vi "Sequence Create PDA Column.vi"(8 "error in (no error)":errorcluster, 11 "Connection Refnum":T1) -> (0 "error out":errorcluster, 3 "Connection Refnum":T1)   [LabVIEW 2011]
uses:
  SI.LIB/ODBC/SQL Controls/Connection Refnum.ctl
panel:
  out "Possible error out":errorcluster
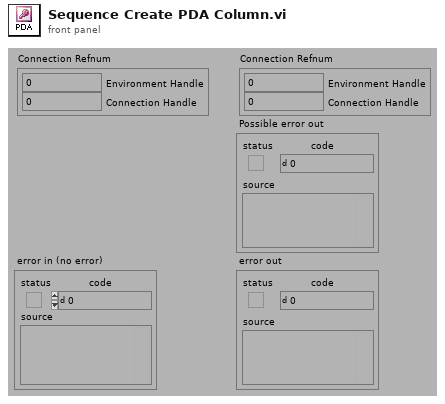
[diagram p1: front panel]
types:
  T1 = typedef "Connection Refnum.ctl" = cluster{"Environment Handle":i32, "Connection Handle":i32}
  T2 = typedef "Statement Refnum.ctl" = cluster{"Statement Handle":i32, "Parameter Number":u16}
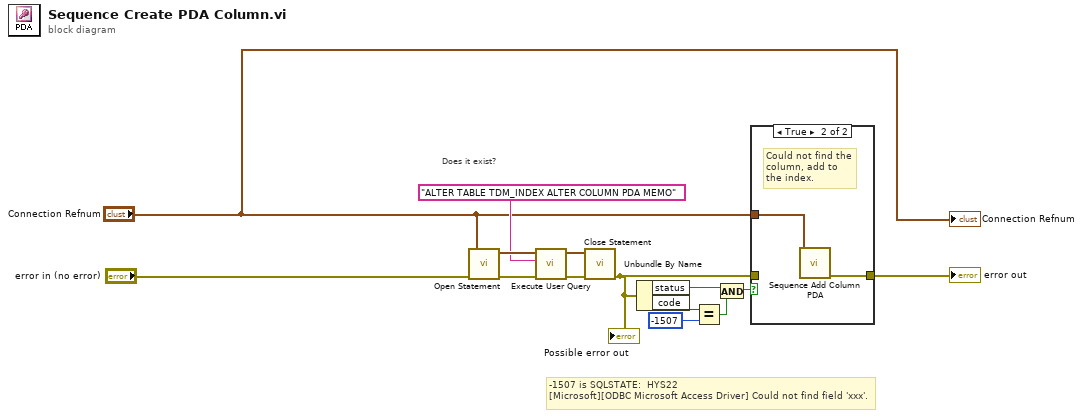
[diagram p0: block diagram]
diagram:
  # "Does it exist?"
  # "-1507 is SQLSTATE:  HYS22\n[Microsoft][ODBC Microsoft Access Driver] Could not find field 'xxx'."
  n1 = call "Open Statement.vi"("error in (no error)"="error in (no error)", "Connection Refnum"="Connection Refnum") -> ("error out"=w13:errorcluster, "Statement Refnum"=w14:T2)  [unwired: 4 out]
  n2 = call "Execute User Query.vi"("error in (no error)"=w13, "User Query"="ALTER TABLE TDM_INDEX ALTER COLUMN PDA MEMO" ("format string"), "Statement Refnum"=w14) -> ("error out"=w12:errorcluster, "Statement Refnum"=w11:T2)  [unwired: 1 in, 2 out]
  n3 = call "Close Statement.vi"("error in (no error)"=w12, "Statement Refnum"=w11) -> ("error out"=w5:errorcluster)  [unwired: 5 out]
  "Possible error out" <- w5
  n4 = Unbundle By Name(w5) -> ("status"=w9:bool, "code"=w8:i32)
  n5 = Equal?(x=w8, y=-1507) -> (x = y?=w7:bool)
  n6 = And(x=w9, y=w7) -> (x .and. y?=w10:bool)
  n7 = case shown="True" w10 {
    tunnel: [w15 w16] -> w3
    tunnel: "Connection Refnum" -> [_ w17]
    tunnel: w5 -> [w15 _]
    frame False {
      # "Column exists"
    }
    frame True {
      # "Could not find the \ncolumn, add to\nthe index."
      n8 = call "Sequence Add Column PDA.vi"("Connection Refnum"=w17) -> ("error out"=w16:errorcluster)  [unwired: 1 in, 9 out]
    }
  }
  "error out" <- w3
  "Connection Refnum" <- "Connection Refnum"
